vi "ImPro - Shadow Adjustment.vi"(8 "error in (no error)":errorcluster, 10 "24-bit pixmap In":u32[][](array[numeric]), 11 "Shadows (%)":dbl) -> (0 "error out":errorcluster, 2 "24-bit pixmap Out":u32[][](array[numeric]), 3 "R 1D Array":u8[](array[numeric]))   [LabVIEW 2023]
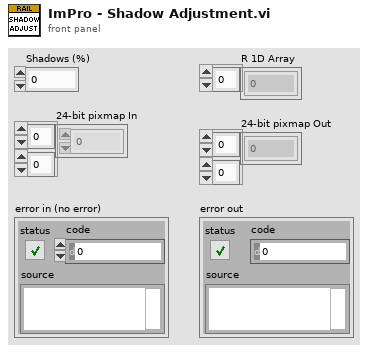
[diagram p1: front panel]
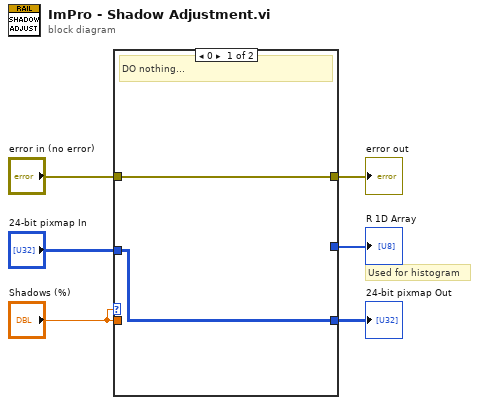
[diagram p0: block diagram]
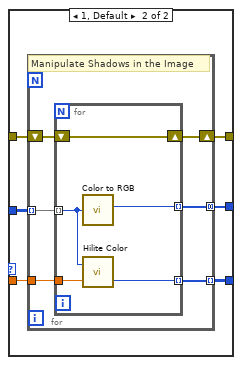
[diagram p2: hidden frame]
diagram:
  # "Used for histogram"
  n1 = case shown="0" "Shadows (%)" {
    tunnel: [w7 w14] -> w6
    tunnel: "error in (no error)" -> [w7 w13]
    tunnel: "Shadows (%)" -> [_ w12]
    tunnel: [w8 w11] -> w4
    tunnel: [_ w10] -> w3
    tunnel: "24-bit pixmap In" -> [w8 w9]
    frame 0 {
      # "DO nothing..."
    }
    frame 1, Default {
      n2 = for {
        tunnel: w9 -> [w18] mode=indexing
        tunnel: w12 -> [w20]
        tunnel: [w19] -> w11 mode=indexing
        tunnel: [w17] -> w10 mode=concatenating
        shift-right: [w15] -> w14
        shift-left: w13 -> [w16]
        # "Manipulate Shadows in the Image"
        n3 = for {
          tunnel: w18 -> [w23] mode=indexing
          tunnel: w20 -> [w25]
          tunnel: [w24] -> w19 mode=indexing
          tunnel: [w22] -> w17 mode=indexing
          shift-right: [w21] -> w15
          shift-left: w16 -> [w21]
          n4 = call <vilib>:"Color to RGB.vi"("Color"=w23) -> ("R"=w22:u8)  [unwired: 3 out]
          n5 = call <vilib>:"Hilite Color.vi"("Percentage(30)"=w25, "Color In"=w23) -> ("Shadow"=w24:u32)  [unwired: 1 out]
        }
      }
    }
  }
  "error out" <- w6
  "24-bit pixmap Out" <- w4
  "R 1D Array" <- w3
